vi "FPGA Main.vi"() -> ()   [LabVIEW 2009]
uses:
  <vilib>/eio/EIONode/EIONode.xnode
  <vilib>/rvi/eio/nirviEIOImplementation/nirviEIOImplementation.xnode
  <vilib>/rvi/eio/common/nirviEmuTemplateMethod_noerrors.vi
  <vilib>/rvi/eio/common/nirviEmuClasses.ctl
panel:
  in  "stop":bool
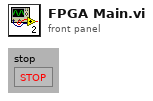
[diagram p1: front panel]
types:
  T1 = typedef "nirviEmuClasses.ctl" = enum16{"IO Read", "IO Write", "Method", "Property Read", "Property Write"}
  T2 = cluster{"x (LIDAR data position)":i16, "y (LIDAR data position) ":i16, "theta  (LIDAR scan position)":u8}
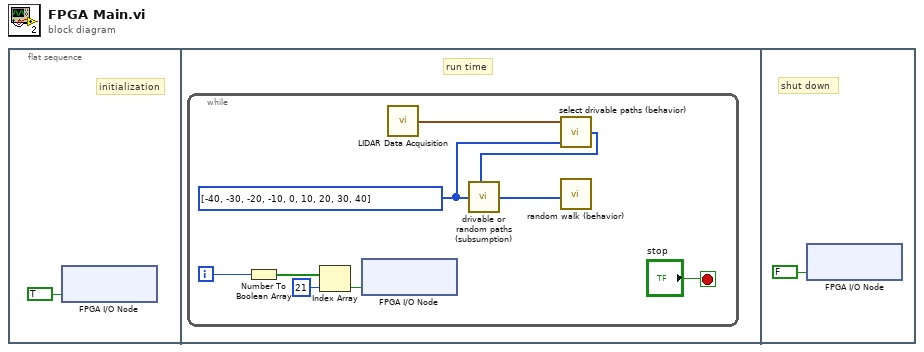
[diagram p0: block diagram]
diagram:
  n1 = flat-sequence {
    frame #0 {
      # "initialization"
      n2 = xnode "FPGA I/O Node"("FPGA LED"=TRUE) -> ()  [unwired: 1 in, 1 out]
    }
    frame #1 {
      # "run time"
      n3 = while {
        i -> [w17]
        stop <- "stop" stop-if-true
        w18 = i8[] [-40, -30, -20, -10, 0, 10, 20, 30, 40]
        n4 = Number To Boolean Array(number=w17) -> (Boolean array=w16:bool[])
        n5 = Index Array(array=w16, index=21) -> (element=w13:bool)
        n6 = xnode "FPGA I/O Node"("FPGA LED"=w13) -> ()  [unwired: 1 in, 1 out]
        n7 = call "LIDAR Data Acquisition.vi"() -> ("LIDAR Data"=w19:T2)  [unwired: 5 in]
        n8 = call "select drivable paths (behavior).vi"("possible drive vectors"=w18, "LIDAR Data"=w19) -> ("driveable drive vectors"=w20:i8[])  [unwired: 3 in]
        n9 = call "drivable or random paths (subsumption).vi"("driveable drive vectors"=w20, "possible drive vectors"=w18) -> ("choosen drive vectors"=w21:i8[])  [unwired: 5 in]
        n10 = call "random walk (behavior).vi"("possible drive vectors"=w21) -> ()  [unwired: 4 in, 1 out]
      }
    }
    frame #2 {
      # "shut down"
      n11 = xnode "FPGA I/O Node"("FPGA LED"=FALSE) -> ()  [unwired: 1 in, 1 out]
    }
  }
